vi "String Ends With.vi"(10 "ends with":string, 11 "string":string) -> (3 "ends with?":bool)   [LabVIEW 2020]
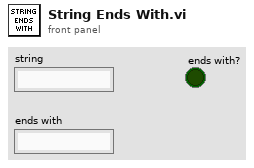
[diagram p1: front panel]
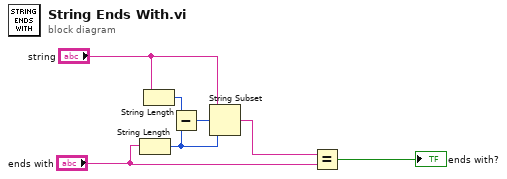
[diagram p0: block diagram]
diagram:
  n1 = String Length(string="ends with") -> (length=w3:i32)
  n2 = String Length(string="string") -> (length=w2:i32)
  n3 = Subtract(x=w2, y=w3) -> (x-y=w4:i32)
  n4 = String Subset(string="string", offset (0)=w4, length (rest)=w3) -> (substring=w5:string)
  n5 = Equal?(x=w5, y="ends with") -> (x = y?=→"ends with?":bool)
